vi "Get APU.vi"(8 "error in (no error)":errorcluster, 11 "APU Node":refnum<k24>) -> (0 "error out":errorcluster, 2 "APU Settings":T1, 3 "APU Node":refnum<k24>)   [LabVIEW 2015, in "Engine Simulation Toolkit SysDef API.lvlib"]
uses:
  Engine Simulation Toolkit SysDef API.lvlib
  NationalInstruments.VeriStand.SystemDefinitionAPI
  APU Settings.ctl
  Shared/Properties.vi
  Shared/Constants and GUIDs.vi
  <vilib>/NI Veristand/Custom Device API/Get Item Property (Double).vi
  <vilib>/NI Veristand/Custom Device Tools/Custom Device Utility Library/NI VeriStand - Search for Item by Name.vi
  <vilib>/NI Veristand/Custom Device API/Get Item Property (Boolean).vi
  Shared/Engine Simulation Toolkit Shared.lvlib
  <vilib>/NI VeriStand/Custom Device API/Custom Device API.lvlib
  <vilib>/NI VeriStand/Custom Device Tools/Custom Device Utility Library/Custom Device Utility Library.lvlib
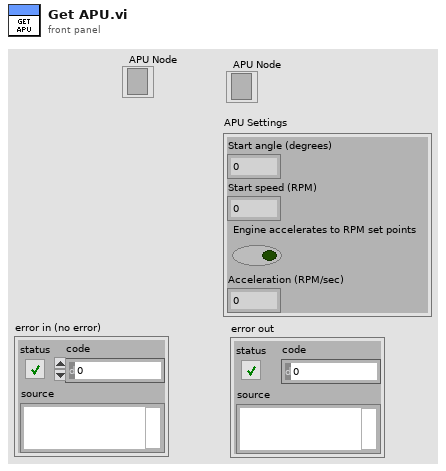
[diagram p1: front panel]
types:
  T1 = typedef "Engine Simulation Toolkit SysDef API.lvlib/APU Settings.ctl" = cluster{"Start angle (degrees)":dbl, "Start speed (RPM)":dbl, "Engine accelerates to RPM set points":bool, "Acceleration (RPM/sec)":dbl}
  T2 = typedef "Engine Simulation Toolkit Shared.lvlib/Channel.ctl" = cluster{"Name":string, "Units":string, "Default":dbl, "Description":string, "Scalable":bool}
  T3 = typedef "Custom Device API.lvlib/Custom Device Item Ref.ctl" = u64
  T4 = typedef "Custom Device API.lvlib/Custom Device Channel.ctl" = cluster{"Type":T5, "Units":string, "Default Value":dbl, "Faultable":bool, "Scalable":bool}
  T5 = typedef "Custom Device API.lvlib/Custom Device Channel Type.ctl" = enum16{"Input", "Output"}
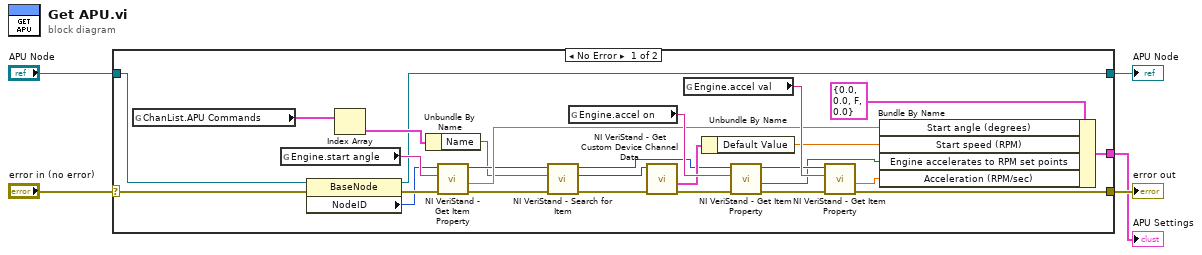
[diagram p0: block diagram]
diagram:
  n1 = case shown="No Error" "error in (no error)" {
    selector: "error in (no error)" -> [w23 w34]
    tunnel: [w28 w34] -> w5
    tunnel: "APU Node" -> [w24 w33]
    tunnel: [w21 w33] -> w2
    tunnel: [w19 _] -> w1
    frame No Error {
      n2 = global read "Constants and GUIDs.vi" "ChanList.APU Commands"() -> (w26:T2[])
      n3 = global read "Properties.vi" "Engine.start angle"() -> (w31:string)
      n4 = property class="BaseNode"(reference=w24, error in=w23) -> (reference out=w21:refnum<k24>, error out=w22:errorcluster, "NodeID"=w20:u64)
      n5 = Index Array(array=w26) -> (element=w27:T2)  [unwired: 1 in]
      n6 = Unbundle By Name(w27) -> ("Name"=w10:string)
      n7 = call-poly <vilib>:"NI VeriStand - Get Item Property.vi"("error in (no error)"=w22, "Property Name"=w31, "Item Ref in"=w20) -> ("error out"=w9:errorcluster, "Value"=w17:dbl, "Item Ref out"=w11:T3)  [unwired: 5 in, 1 out]
      n8 = call-poly <vilib>:"NI VeriStand - Search for Item.vi"("error in"=w9, "Item Name"=w10, "Section Ref in"=w11) -> ("error out"=w8:errorcluster, "Item Ref"=w7:T3, "Section Ref out"=w6:T3)  [unwired: 5 in, 1 out]
      n9 = global read "Properties.vi" "Engine.accel on"() -> (w32:string)
      n10 = call <vilib>:"NI VeriStand - Get Custom Device Channel Data.vi"("error in (no error)"=w8, "Channel Ref in"=w7) -> ("error out"=w15:errorcluster, "Channel"=w14:T4)  [unwired: 4 in, 4 out]
      n11 = global read "Properties.vi" "Engine.accel val"() -> (w30:string)
      n12 = Unbundle By Name(w14) -> ("Default Value"=w13:dbl)
      n13 = call-poly <vilib>:"NI VeriStand - Get Item Property.vi"("error in (no error)"=w15, "Property Name"=w32, "Item Ref in"=w6) -> ("error out"=w29:errorcluster, "Value"=w16:bool, "Item Ref out"=w25:T3)  [unwired: 5 in, 1 out]
      n14 = call-poly <vilib>:"NI VeriStand - Get Item Property.vi"("error in (no error)"=w29, "Property Name"=w30, "Item Ref in"=w25) -> ("error out"=w28:errorcluster, "Value"=w12:dbl)  [unwired: 5 in, 2 out]
      n15 = Bundle By Name(cluster=T1 {"Start angle (degrees)"=0.0, "Start speed (RPM)"=0.0, "Engine accelerates to RPM set points"=FALSE, "Acceleration (RPM/sec)"=0.0} ("APU Settings"), "Start angle (degrees)"=w17, "Start speed (RPM)"=w13, "Engine accelerates to RPM set points"=w16, "Acceleration (RPM/sec)"=w12) -> (w19:T1)
    }
    frame Error {
    }
  }
  "error out" <- w5
  "APU Node" <- w2
  "APU Settings" <- w1
